vi "TEST_subVI.vi"(10 "number":i32, 11 "input":dbl) -> ()   [LabVIEW 2023]
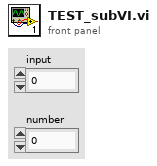
[diagram p1: front panel]
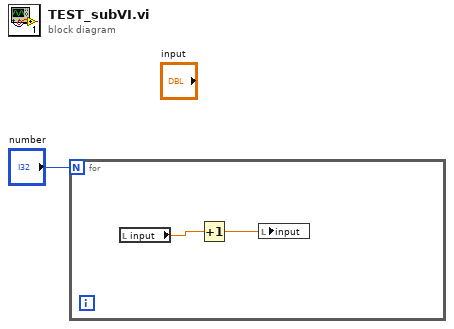
[diagram p0: block diagram]
diagram:
  n1 = for {
    N: "number" -> [_]
    n2 = local read "input"() -> (w3:dbl)
    n3 = Increment(x=w3) -> (x+1=w2:dbl)
    n4 = local write "input"(w2) -> ()
  }
